vi "emotion_recognize.vi"() -> ()   [LabVIEW 2014]
uses:
  <vilib>/sound2/lvsound2.llb/Sampling Mode.ctl
  <vilib>/sound2/lvsound2.llb/Sound Data Format.ctl
  <vilib>/sound2/lvsound2.llb/Sound File Write Open.vi
  <vilib>/sound2/lvsound2.llb/Sound Input Read (DBL).vi
  <vilib>/sound2/lvsound2.llb/Sound File Write (DBL).vi
  <vilib>/sound2/lvsound2.llb/Sound File Info (path).vi
  <vilib>/sound2/lvsound2.llb/Sound File Read Open.vi
  <vilib>/sound2/lvsound2.llb/Sound File Read (DBL).vi
  <vilib>/vi.lib/Utility/file.llb/Write To Spreadsheet File (DBL).vi
  <vilib>/vi.lib/Utility/file.llb/Read From Spreadsheet File (DBL).vi
panel:
  in  "?":bool
  in  "开始识别":bool
  in  "停止":bool
  in  "开始训练":bool
  in  "特征提取":bool
  in  "?":bool
  in  "模型选择":u16(ring) items=["使用内置训练数据", "手动选择训练数据"]
  in  "感情种类":u16(ring) items=["0", "1", "2", "3", "4", "5", "6"]
  in  "训练次数":dbl
  in  "输入数据":path
  in  "启动测试":bool
  in  "结束测试":bool
  in  "path":path=path "D:/sound/1.wav" caption="存储路径"
  in  "录音播放":bool
  in  "循环次数":i32=2
  in  "播放时间":u32=10
  in  "录音时间":u32=10
  out "error out":errorcluster caption="错误输出"
  in  "选项卡控件":enum32{"录音&播放", "特征提取", "训练", "识别"}(tab)
  out "波形图 2":waveform(dbl)[](graph)
  out "?":waveform(dbl)[](graph)
  out "?":string
  out "?":string
  out "结果":string
  # "录音&播放"
  # "特征提取"
  # "训练数据"
  # "情感识别"
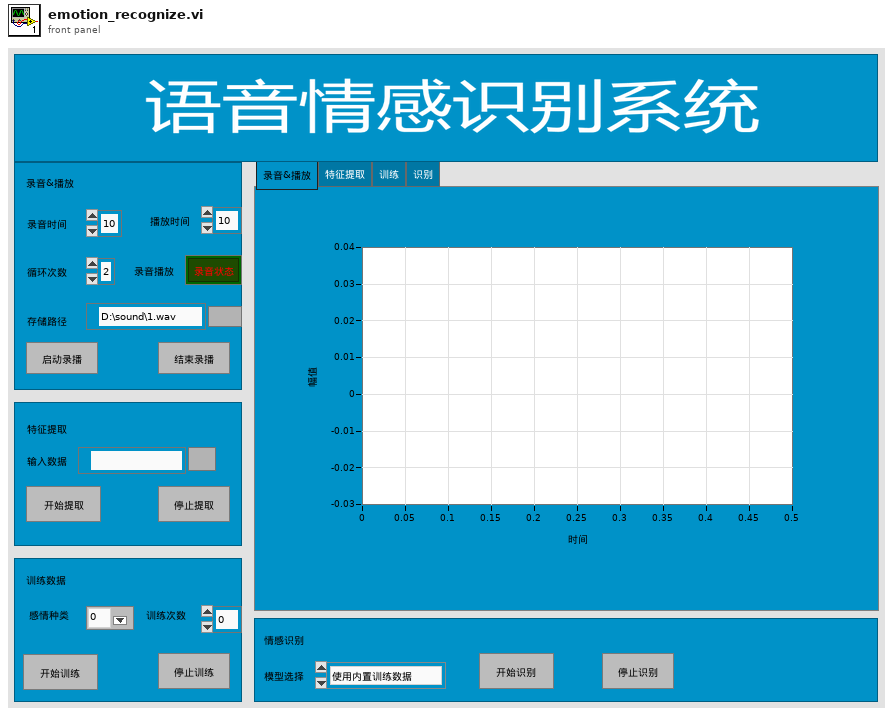
[diagram p1: front panel]
types:
  T1 = typedef "Sound Data Format.ctl" = cluster{"sample rate (S/s)":dbl, "number of channels":i32, "bits per sample":i32}
  T2 = typedef "Sampling Mode.ctl" = i32
  T3 = typedef "Sound Input Task ID.ctl" = u32
  T4 = typedef "Sound File Refnum.ctl" = refnum<file>
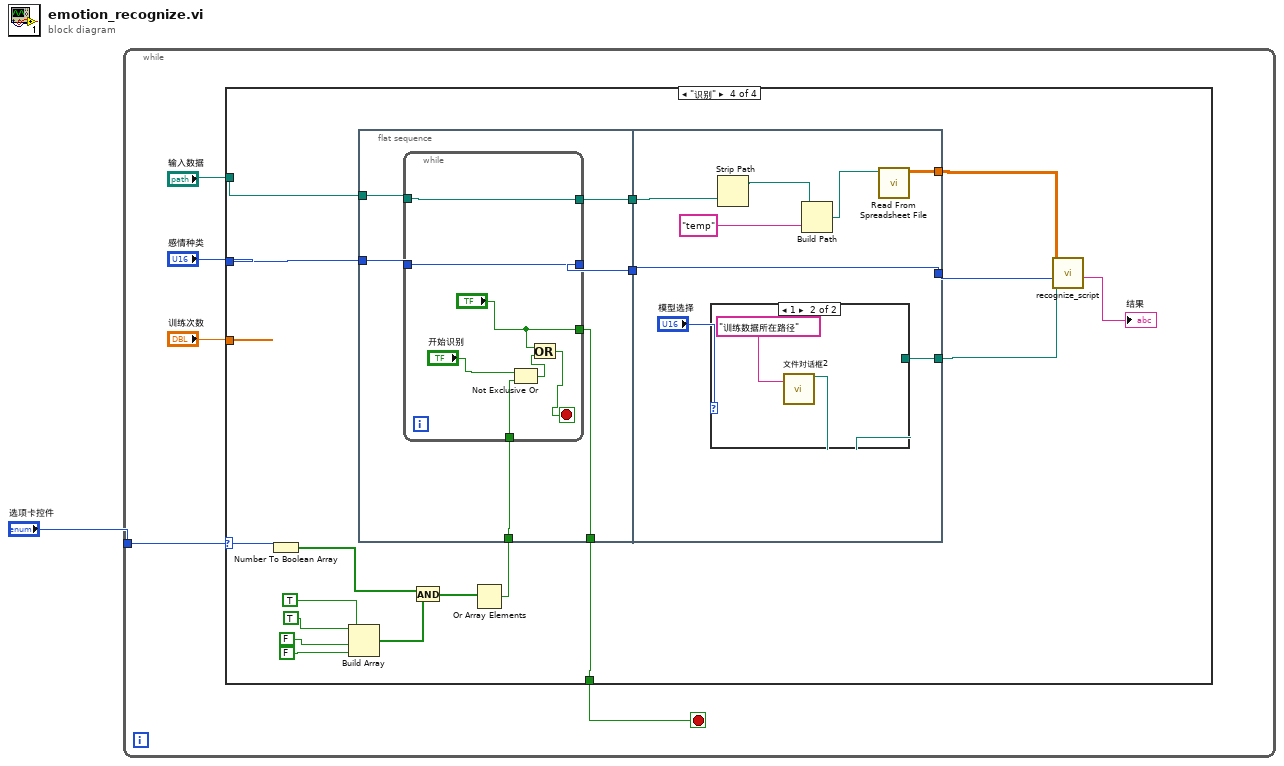
[diagram p0: block diagram]
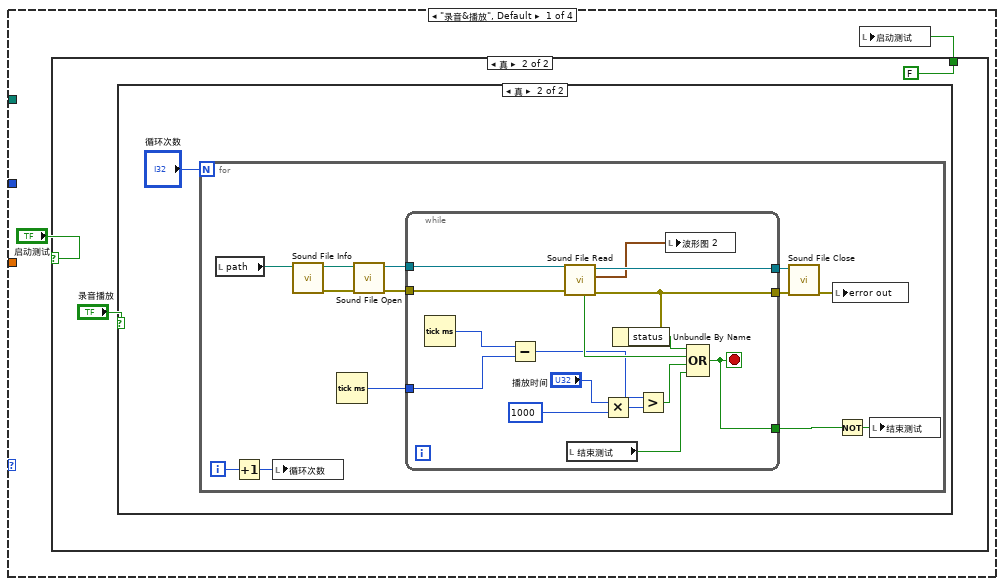
[diagram p2: hidden frame]
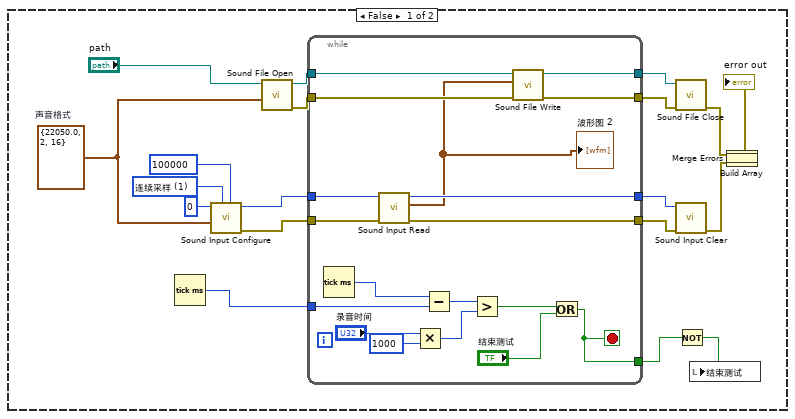
[diagram p4: hidden frame]
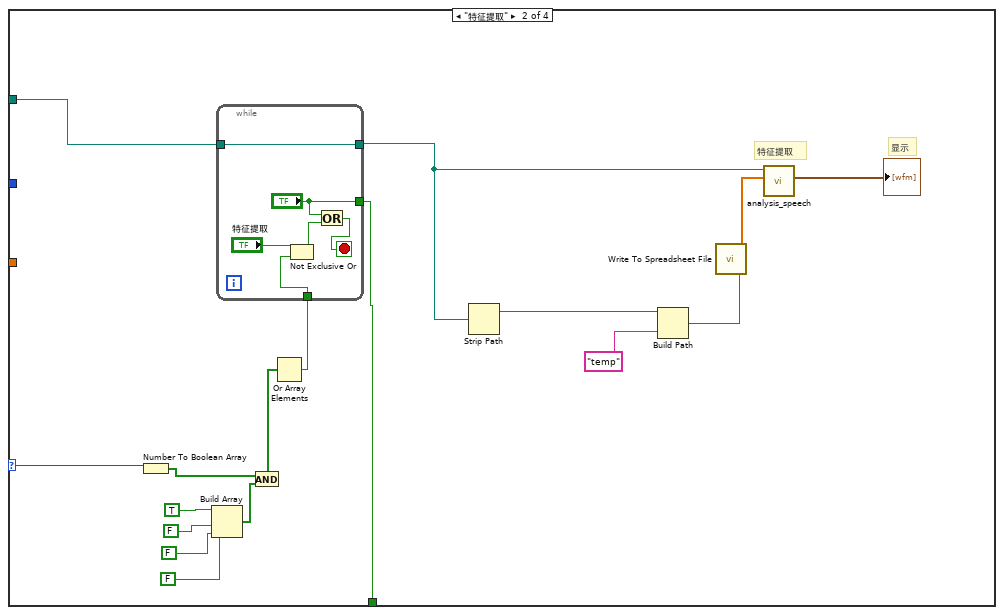
[diagram p5: hidden frame]
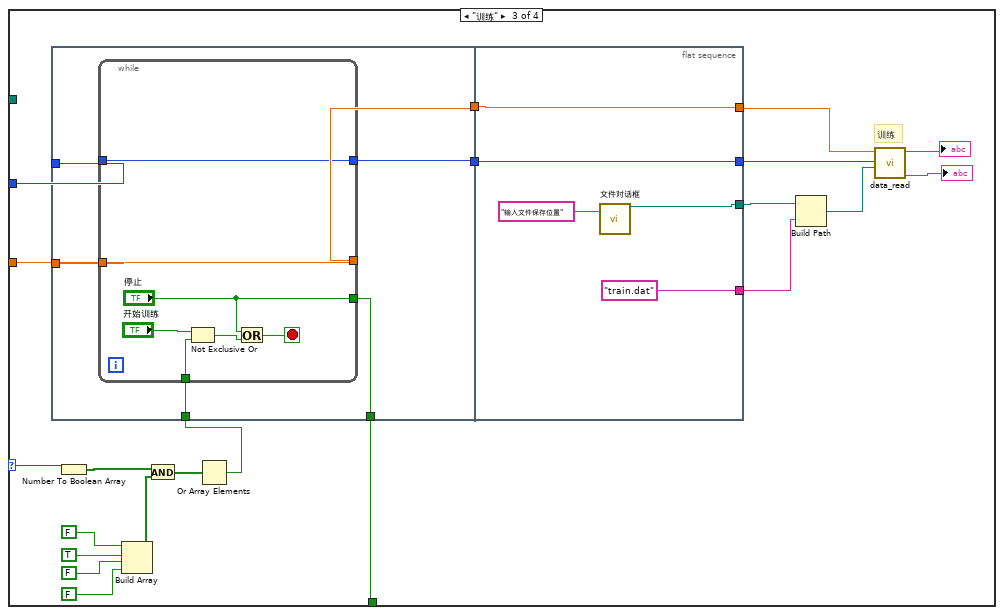
[diagram p6: hidden frame]
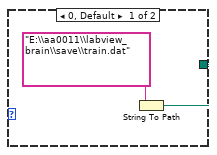
[diagram p7: hidden frame]
diagram:
  n1 = while {
    tunnel: "选项卡控件" -> [w3]
    stop <- w2 stop-if-true
    n2 = case "条件结构" shown="\"识别\"" w3 {
      selector: w3 -> [_ w84 w112 w154]
      tunnel: "训练次数" -> [_ _ w120 _]
      tunnel: "感情种类" -> [_ _ w122 w156]
      tunnel: "输入数据" -> [_ w80 _ w158]
      tunnel: [_ w79 w102 w141] -> w2
      frame "录音&播放", Default {
        n3 = case shown="真" "启动测试" {
          tunnel: [_ FALSE] -> w8
          frame False {
          }
          frame True {
            n4 = case shown="真" "录音播放" {
              frame False {
                w27 = T1 {"sample rate (S/s)"=22050.0, "number of channels"=2, "bits per sample"=16}  # 声音格式
                w28 = T2 1 items=["有限采样", "连续采样"] ("采集模式")
                n5 = Tick Count (ms)() -> (millisecond timer value=w19:u32)
                n6 = call <vilib>:"Sound Input Configure.vi"("number of samples/ch"=100000 ("采集点数"), "sample mode"=w28, "sound format"=w27, "device ID"=u32 0 ("设备号")) -> ("error out"=w24:errorcluster, "task ID"=w25:T3)  [unwired: 1 in, 5 out]
                n7 = call-poly <vilib>:"Sound File Open.vi"("sound format"=w27, "path"="path") -> ("error out"=w17:errorcluster, "sound file refnum"=w23:T4)  [unwired: 1 in, 7 out]
                n8 = while {
                  tunnel: w25 -> [w48]
                  tunnel: w24 -> [w47]
                  tunnel: w23 -> [w46]
                  tunnel: [w45] -> w22
                  tunnel: [w33] -> w21
                  tunnel: [w44] -> w20
                  tunnel: w19 -> [w42]
                  tunnel: [w35] -> w18
                  tunnel: w17 -> [w34]
                  tunnel: [w32] -> w13
                  stop <- w32 stop-if-true
                  n9 = Tick Count (ms)() -> (millisecond timer value=w43:u32)
                  n10 = call-poly <vilib>:"Sound Input Read.vi"("error in (no error)"=w47, "task ID"=w48) -> ("error out"=w33:errorcluster, "data"=w31:waveform(dbl)[], "task ID out"=w45:T3)  [unwired: 2 in, 5 out]
                  "波形图 2" <- w31
                  n11 = Multiply(x="录音时间", y=u32 1000) -> (x*y=w37:u32)
                  n12 = Subtract(x=w43, y=w42) -> (x-y=w41:u32)
                  n13 = Greater?(x=w41, y=w37) -> (0:w39:bool)
                  n14 = call-poly <vilib>:"Sound File Write.vi"("error in (no error)"=w34, "data"=w31, "sound file refnum"=w46) -> ("error out"=w35:errorcluster, "sound file refnum out"=w44:T4)  [unwired: 7 out]
                  n15 = Or(x=w39, y="结束测试") -> (x .or. y?=w32:bool)
                }
                n16 = call <vilib>:"Sound File Close.vi"("error in (no error)"=w18, "sound file refnum"=w20) -> ("error out"=w16:errorcluster)  [unwired: 9 out]
                n17 = call <vilib>:"Sound Input Clear.vi"("error in (no error)"=w21, "task ID"=w22) -> ("error out"=w15:errorcluster)  [unwired: 9 out]
                n18 = Not(x=w13) -> (.not. x?=w12:bool)
                n19 = local write "结束测试"(w12) -> ()
                n20 = Build Array(w16, w15) -> (w11:errorcluster[])
                n21 = Merge Errors(w11) -> (→"error out":errorcluster)
              }
              frame True {
                n22 = for {
                  N: "循环次数" -> [_]
                  i -> [w62]
                  n23 = local read "path"() -> (w60:path)
                  n24 = Increment(x=w62) -> (x+1=w61:i32)
                  n25 = local write "循环次数"(w61) -> ()
                  n26 = call-poly <vilib>:"Sound File Info.vi"("path"=w60) -> ("error out"=w59:errorcluster, "path out"=w58:path)  [unwired: 7 in, 2 out]
                  n27 = Tick Count (ms)() -> (millisecond timer value=w52:u32)
                  n28 = call-poly <vilib>:"Sound File Open.vi"("error in (no error)"=w59, "path"=w58) -> ("error out"=w56:errorcluster, "sound file refnum"=w57:T4)  [unwired: 8 in]
                  n29 = while {
                    tunnel: w57 -> [w78]
                    tunnel: w56 -> [w77]
                    tunnel: [w74] -> w55
                    tunnel: [w76] -> w54
                    tunnel: w52 -> [w72]
                    tunnel: [w67] -> w51
                    stop <- w67 stop-if-true
                    n30 = Tick Count (ms)() -> (millisecond timer value=w73:u32)
                    n31 = Subtract(x=w73, y=w72) -> (x-y=w71:u32)
                    n32 = call-poly <vilib>:"Sound File Read.vi"("error in (no error)"=w77, "sound file refnum"=w78) -> ("error out"=w74:errorcluster, "data"=w63:waveform(dbl)[], "sound file refnum out"=w76:T4, "end of file?"=w75:bool)  [unwired: 5 in, 1 out]
                    n33 = local read "结束测试"() -> (w68:bool)
                    n34 = Multiply(x="播放时间", y=u32 1000) -> (x*y=w66:u32)
                    n35 = Unbundle By Name(w74) -> ("status"=w64:bool)
                    n36 = Greater?(x=w71, y=w66) -> (0:w69:bool)
                    n37 = local write "波形图 2"(w63) -> ()
                    n38 = Compound Arithmetic op=OR(w64, w75, w69, w68) -> (w67:bool)
                  }
                  n39 = call <vilib>:"Sound File Close.vi"("error in (no error)"=w55, "sound file refnum"=w54) -> ("error out"=w53:errorcluster)  [unwired: 9 in]
                  n40 = local write "error out"(w53) -> ()
                  n41 = Not(x=w51) -> (.not. x?=w50:bool)
                  n42 = local write "结束测试"(w50) -> ()
                }
              }
            }
          }
        }
        n43 = local write "启动测试"(w8) -> ()
      }
      frame "特征提取" {
        # "显示"
        # "特征提取"
        n44 = Number To Boolean Array(number=w84) -> (Boolean array=w87:bool[])
        n45 = Build Array(TRUE, FALSE, FALSE, FALSE) -> (w86:bool[])
        n46 = And(x=w87, y=w86) -> (x .and. y?=w85:bool[])
        n47 = Or Array Elements(Boolean array=w85) -> (logical OR=w83:bool)
        n48 = while {
          tunnel: w80 -> [w101]
          tunnel: [w101] -> w91
          tunnel: w83 -> [w100]
          tunnel: ["?"] -> w79
          stop <- w98 stop-if-true
          n49 = Not Exclusive Or(1:w100, 2:"特征提取") -> (0:w99:bool)
          n50 = Or(x="?", y=w99) -> (x .or. y?=w98:bool)
        }
        n51 = Strip Path(path=w91) -> (stripped path=w94:path)  [unwired: 1 out]
        n52 = Build Path(base path=w94, name or relative path="temp") -> (appended path=w92:path)
        n53 = call "analysis_speech.vi"("文件路径（使用对话框）"=w91) -> ("数组"=w95:dbl[], "波形图表"=→"?":waveform(dbl)[])  [unwired: 9 in]
        n54 = call-poly <vilib>:"Write To Spreadsheet File.vi"("1D data"=w95, "file path (dialog if empty)"=w92) -> ()  [unwired: 6 in, 1 out]
      }
      frame "训练" {
        # "训练"
        n55 = flat-sequence {
          tunnel: w122 -> [w128]
          tunnel: w120 -> [w126]
          tunnel: w111 -> [w124]
          tunnel: [w127] -> w108
          tunnel: [w125] -> w107
          tunnel: [w123] -> w102
          tunnel: [w139] -> w119
          tunnel: [w140] -> w121
          tunnel: w108 -> [w140]
          tunnel: w107 -> [w139]
          tunnel: [w138] -> w106
          tunnel: ["train.dat"] -> w105
          frame #0 {
            n56 = while {
              tunnel: w128 -> [w135]
              tunnel: [w135] -> w127
              tunnel: w126 -> [w134]
              tunnel: [w134] -> w125
              tunnel: w124 -> [w133]
              tunnel: ["停止"] -> w123
              stop <- w131 stop-if-true
              n57 = Not Exclusive Or(1:w133, 2:"开始训练") -> (0:w132:bool)
              n58 = Or(x="停止", y=w132) -> (x .or. y?=w131:bool)
            }
          }
          frame #1 {
            n59 = call "文件对话框"("prompt"="输入文件保存位置") -> ("selected path"=w138:path)  [unwired: 11 in, 3 out]
          }
        }
        n60 = Number To Boolean Array(number=w112) -> (Boolean array=w114:bool[])
        n61 = Build Array(FALSE, TRUE, FALSE, FALSE) -> (w113:bool[])
        n62 = And(x=w114, y=w113) -> (x .and. y?=w110:bool[])
        n63 = Or Array Elements(Boolean array=w110) -> (logical OR=w111:bool)
        n64 = Build Path(base path=w106, name or relative path=w105) -> (appended path=w109:path)
        n65 = call "data_read.vi"("路径"=w109, "感情数目"=w121, "训练次数"=w119) -> ("字符串 2"=→"?":string, "字符串"=→"?":string)  [unwired: 6 in, 1 out]
      }
      frame "识别" {
        n66 = Number To Boolean Array(number=w154) -> (Boolean array=w148:bool[])
        n67 = Build Array(TRUE, TRUE, FALSE, FALSE) -> (w147:bool[])
        n68 = flat-sequence {
          tunnel: w158 -> [w164]
          tunnel: w156 -> [w162]
          tunnel: w153 -> [w160]
          tunnel: [w163] -> w145
          tunnel: [w161] -> w144
          tunnel: [w159] -> w141
          tunnel: [w179] -> w155
          tunnel: w145 -> [w178]
          tunnel: w144 -> [w179]
          tunnel: [w174] -> w143
          tunnel: [w172] -> w142
          frame #0 {
            n69 = while {
              tunnel: w164 -> [w171]
              tunnel: [w171] -> w163
              tunnel: w162 -> [w170]
              tunnel: [w170] -> w161
              tunnel: w160 -> [w169]
              tunnel: ["?"] -> w159
              stop <- w168 stop-if-true
              n70 = Not Exclusive Or(1:w169, 2:"开始识别") -> (0:w167:bool)
              n71 = Or(x="?", y=w167) -> (x .or. y?=w168:bool)
            }
          }
          frame #1 {
            n72 = case shown="1" "模型选择" {
              tunnel: [w180 w182] -> w172
              frame 0, Default {
                n73 = String To Path(string="E:\\aa0011\\labview_brain\\save\\train.dat") -> (path=w180:path)
              }
              frame 1 {
                n74 = call "文件对话框2"("prompt"="训练数据所在路径") -> ("selected path"=w182:path)  [unwired: 11 in, 3 out]
              }
            }
            n75 = Strip Path(path=w178) -> (stripped path=w177:path)  [unwired: 1 out]
            n76 = Build Path(base path=w177, name or relative path="temp") -> (appended path=w175:path)
            n77 = call-poly <vilib>:"Read From Spreadsheet File.vi"("file path (dialog if empty)"=w175) -> ("all rows"=w174:dbl[][])  [unwired: 6 in, 4 out]
          }
        }
        n78 = And(x=w148, y=w147) -> (x .and. y?=w146:bool[])
        n79 = Or Array Elements(Boolean array=w146) -> (logical OR=w153:bool)
        n80 = call "recognize_script.vi"("模板地址"=w142, "识别数据特征"=w143, "选择感情数"=w155) -> ("结果"=→"结果":string)  [unwired: 6 in, 1 out]
      }
    }
  }
